vi "SubPanel_DataCollection_Rev11_v8.vi"(0 "DCPowerInformationClusterArray_Input":T2(array[cluster]), 1 "VISAPowerInfoInputArray":T7(array[cluster]), 2 "Run Data SubPanel Input":T6, 3 "RF Block Parameters":T5, 4 "Oscilloscope Info Array":T4(array[cluster]) {"vertical coupling" items=["AC", "DC", "Ground"]}, 6 "New Run?":bool, 7 "error in":errorcluster) -> (16 "data going into the binary file":T1, 20 "DCPowerInformationClusterArray_Output":T2(array[cluster]), 21 "VISAPowerInfoInputOutput":T7(array[cluster]), 22 "Run Data SubPanel Output":T6, 23 "RF Block Parameters Output":T5, 24 "Oscilloscope Info Array Output":T4(array[cluster]) {"vertical coupling" items=["AC", "DC", "Ground"]}, 25 "Reinitialize?":bool, 26 "Data Was Collected?":bool, 27 "error out":errorcluster)   [LabVIEW 2019]
uses:
  Controls/QueueDataControl.ctl
  Controls/DataBlockControl.ctl
  Controls/QueueDataControl_V2.ctl
  <vilib>/Analysis/NI_AALBase.lvlib
  Controls/QueueDataControl_V3.ctl
  <vilib>/Analysis/1siggen.llb/Ramp Pattern by Delta.vi
  <vilib>/Utility/file.llb/Write Delimited Spreadsheet (string).vi
  Controls/RFBlockControl.ctl
  <instrlib>/niScope/Controls/niScope vertical coupling.ctl
panel:
  out "DCPowerInfoArray":string[][](array[string])
  out "Array":string[][][](array[string])
  out "Current Measurements":cluster{dbl[], dbl[]}[](graph)
  out "Voltage Measurements":cluster{dbl[], dbl[]}[](graph)
  out "DCPowerInformationClusterArray_Input 2":T2(array[cluster])
  out "Exiting":bool
  out "Full Run Information":string
  out "Ready For Next Run?":bool
  in  "Next Run":bool
  out "Latchup Output Data":dbl[][](array[numeric])
  out "Recording Data":bool
  out "Current 2":waveform(dbl)[](graph)
  out "Voltage 2":waveform(dbl)[](graph)
  out "Current":waveform(dbl)[](graph)
  out "Voltage":waveform(dbl)[](graph)
  in  "End Collecting":bool
  in  "Record Data Toggle":bool
  out "error of collection":errorcluster
  in  "force exit SubVI":bool
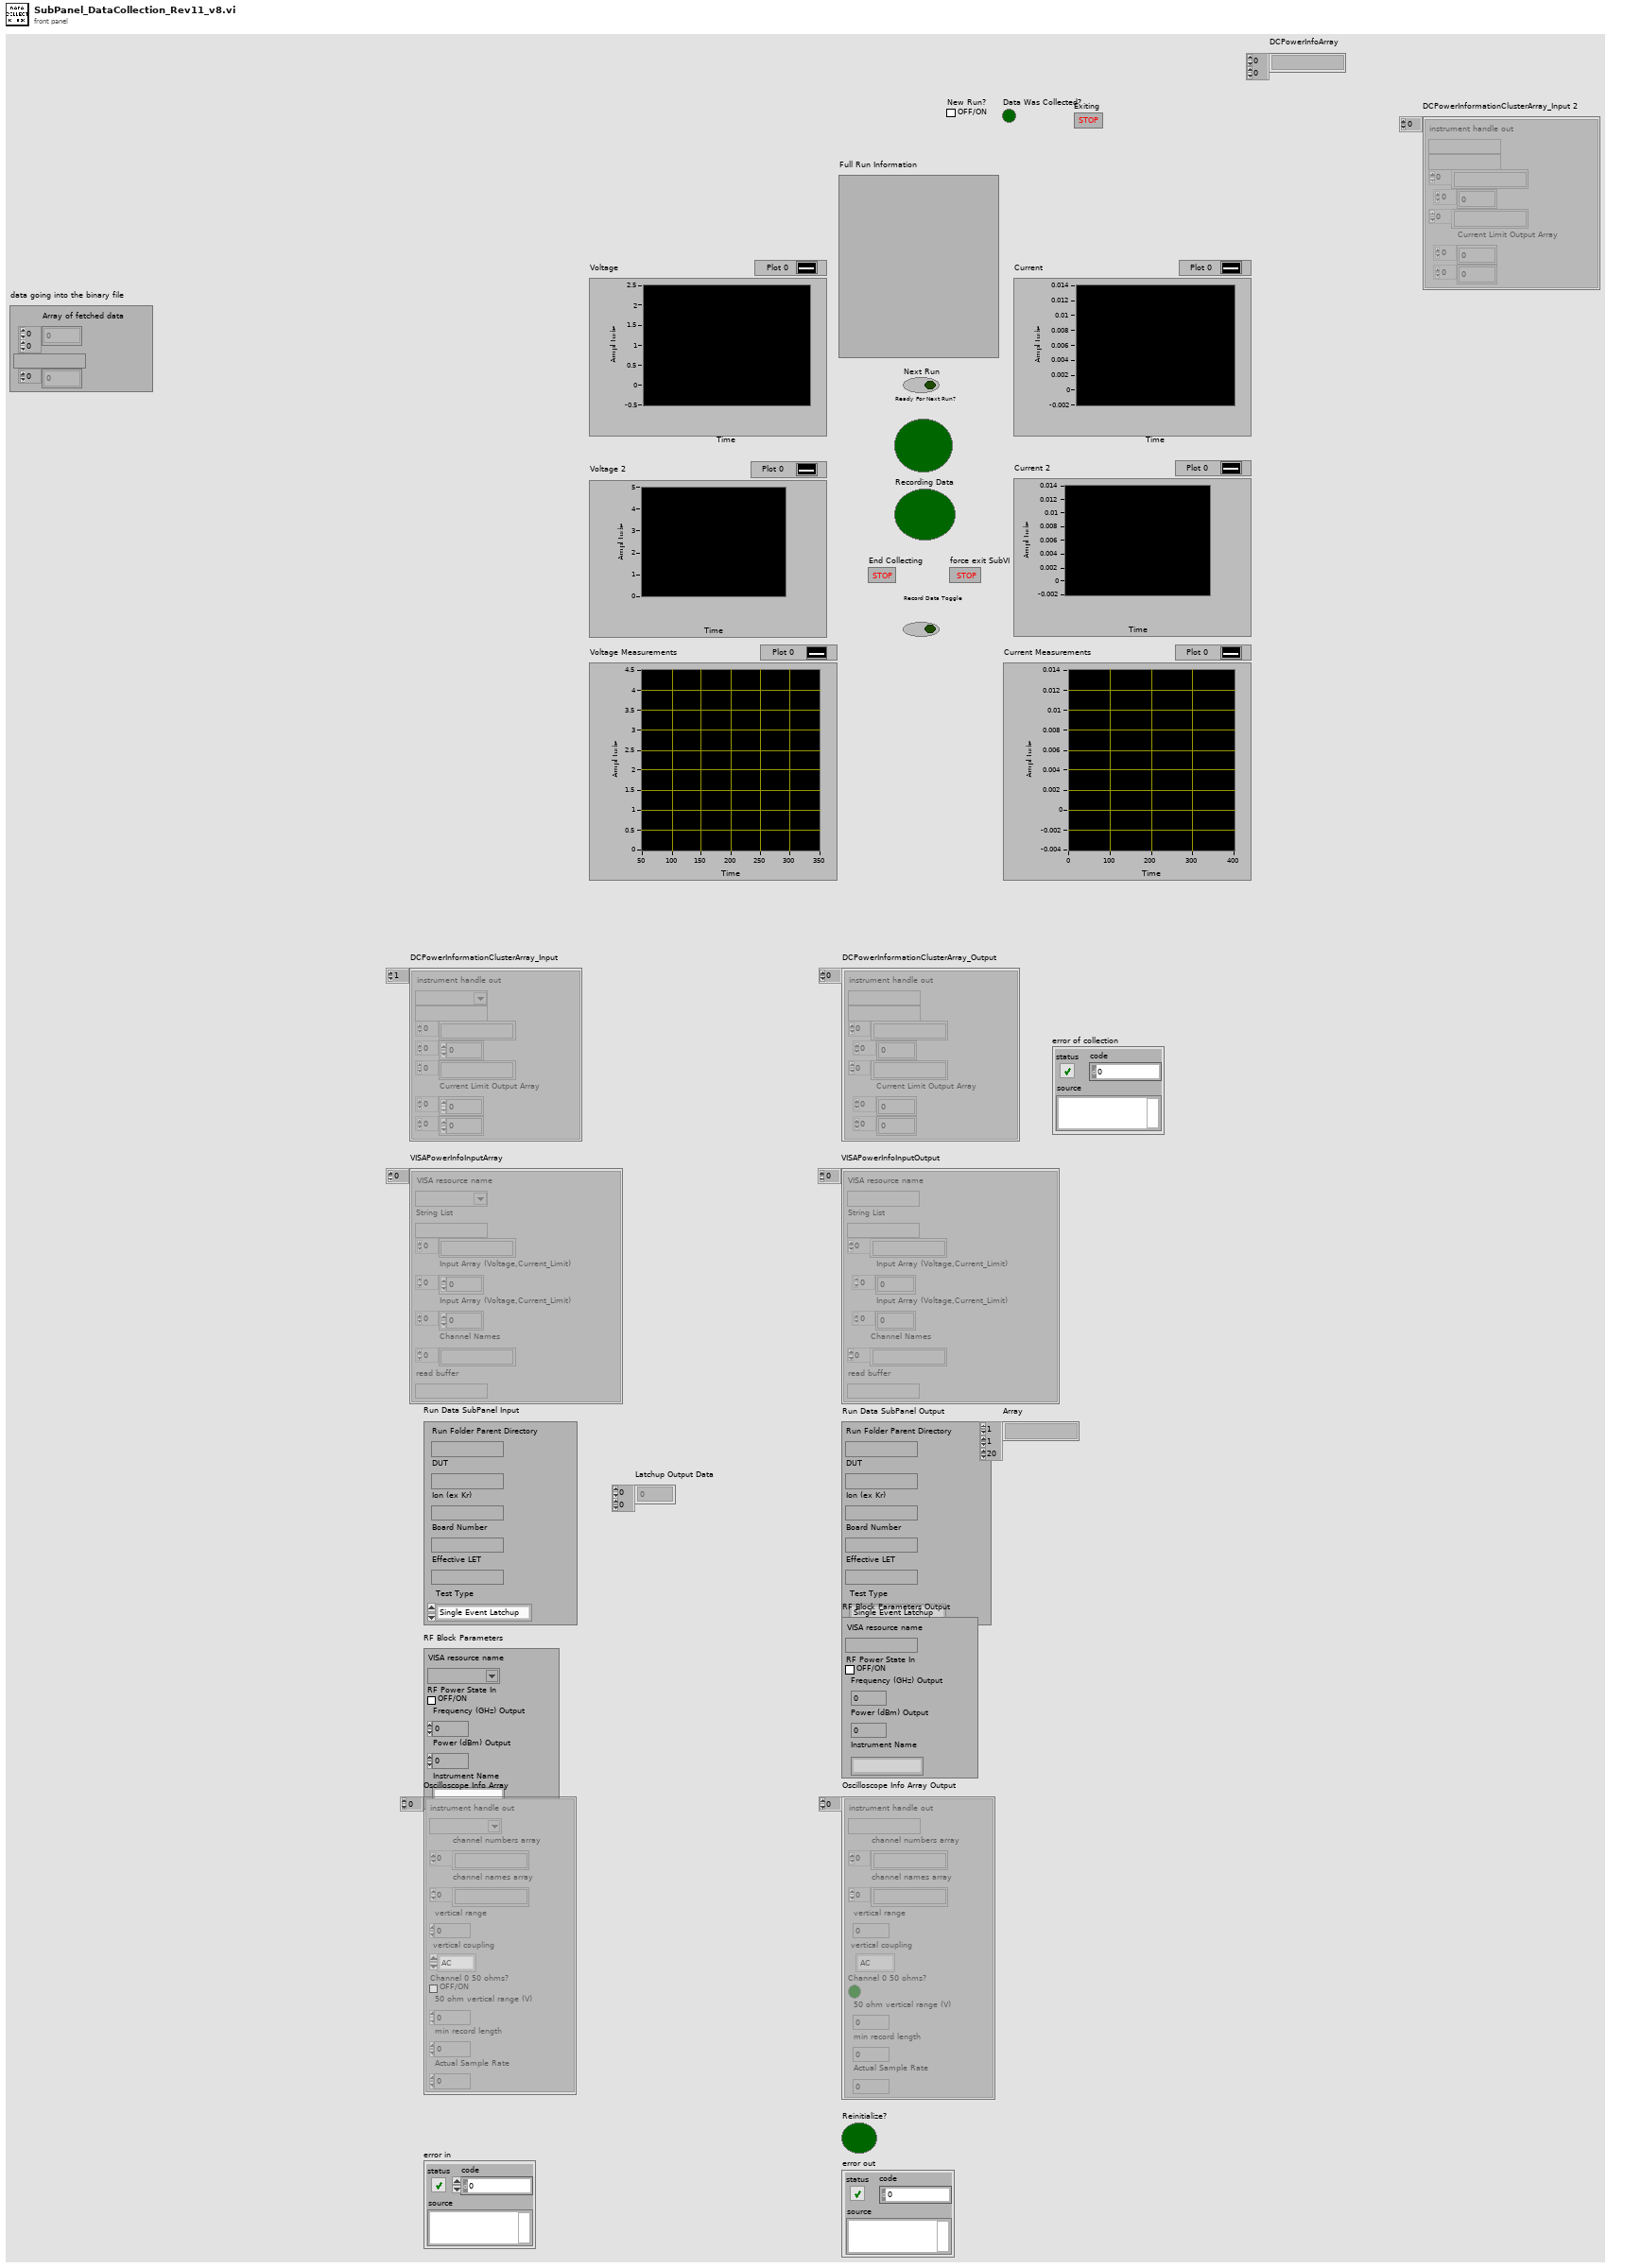
[diagram p1: front panel]
types:
  T1 = cluster{"Array of fetched data":dbl[][], string, i32[]}
  T2 = cluster{"instrument handle out":refnum<k15>, string, string[], dbl[], string[], "Current Limit Output Array":dbl[], dbl[]}[]
  T3 = typedef "niScope vertical coupling.ctl" = i32
  T4 = cluster{"instrument handle out":refnum<k15>, "channel numbers array":string[], "channel names array":string[], "vertical range":dbl, "vertical coupling":T3, "Channel 0 50 ohms?":bool, "50 ohm vertical range (V)":dbl, "min record length":i32, "Actual Sample Rate":dbl}[]
  T5 = typedef "RFBlockControl.ctl" = cluster{"VISA resource name":refnum<visa-resource-name>, "RF Power State In":bool, "Frequency (GHz) Output":dbl, "Power (dBm) Output":dbl, "Instrument Name":string}
  T6 = typedef "DataBlockControl.ctl" = cluster{"Run Folder Parent Directory":path, "DUT":string, "Ion (ex Kr)":string, "Board Number":string, "Effective LET":string, "Test Type":enum16{"Single Event Latchup", "Single Event Transient", "Single Event Upset"}}
  T7 = cluster{"VISA resource name":refnum<visa-resource-name>, "String List":string, string[], "Input Array (Voltage,Current_Limit)":dbl[], "Input Array (Voltage,Current_Limit)":dbl[], "Channel Names":string[], "read buffer":string}[]
  T8 = typedef "QueueDataControl_V3.ctl" = cluster{"Array of fetched data":dbl[][][], "Channel Names Array":string[], "Voltage Waveform Array":waveform(dbl)[], "Current Waveform Array":waveform(dbl)[], "Resetting Time":timestamp, "Beam Logic":dbl}
  T9 = typedef "QueueDataControl_V2.ctl" = cluster{"Time Stamp Array":timestamp[], "Initial Time":timestamp, "dt measurement array":dbl[], "samples per capture":i32[], "voltage measurements":dbl[][], "current measurements":dbl[][]}
  T10 = cluster{"IVI Refnum out":refnum<k15>, string, "voltage level channel 23":dbl, "Channel Name 23":string, "Current Limit":dbl, "Measure Record dt":dbl, string}[]
  T11 = cluster{"created path array":path[], "DCPowerInformation_byChannel":cluster{"IVI Refnum out":refnum<k15>, string, "voltage level channel 23":dbl, "Channel Name 23":string, "Current Limit":dbl, "Measure Record dt":dbl, string}[], string[]}
  T12 = typedef "QueueDataControl.ctl" = cluster{"Rolling Timer":timestamp, "Initial Time":timestamp, "dt between samples":dbl[], "number of samples per fetch":i32[], "voltage measurements":dbl[][], "current measurements":dbl[][]}
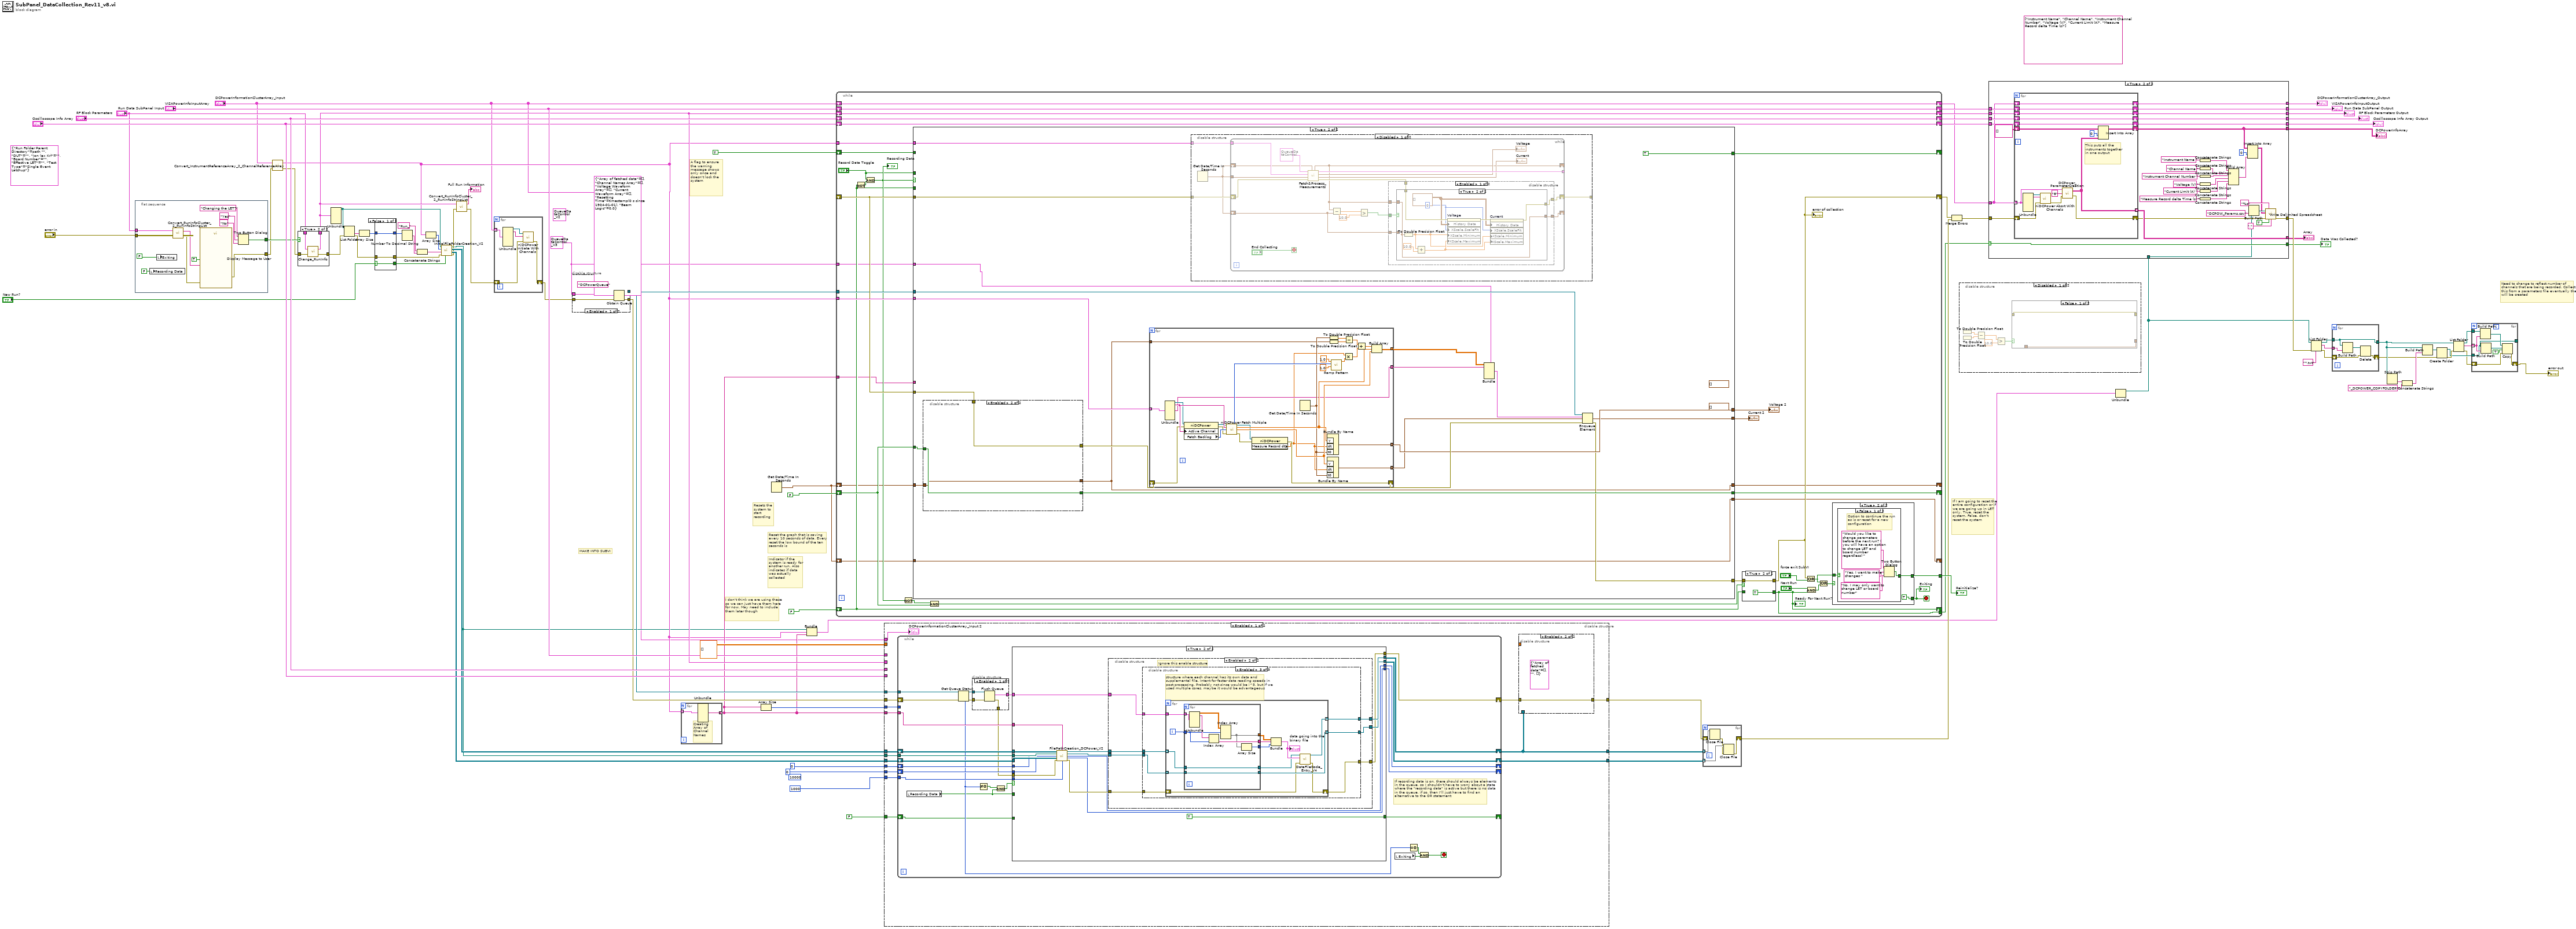
[diagram p0: block diagram]
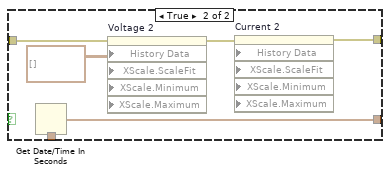
[diagram p2: hidden frame]
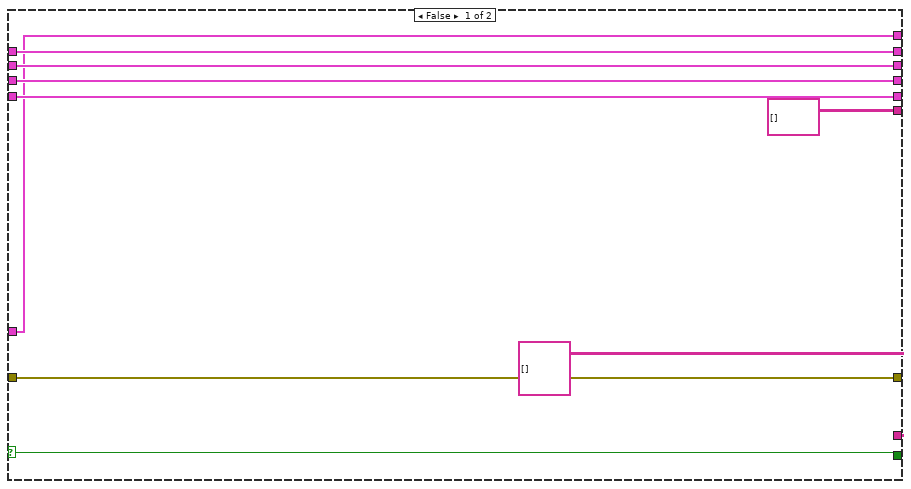
[diagram p4: hidden frame]
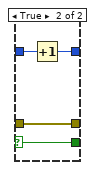
[diagram p5: hidden frame]
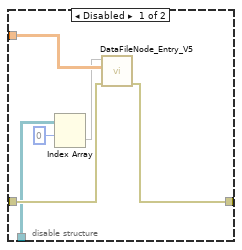
[diagram p8: hidden frame]
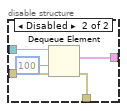
[diagram p9: hidden frame]
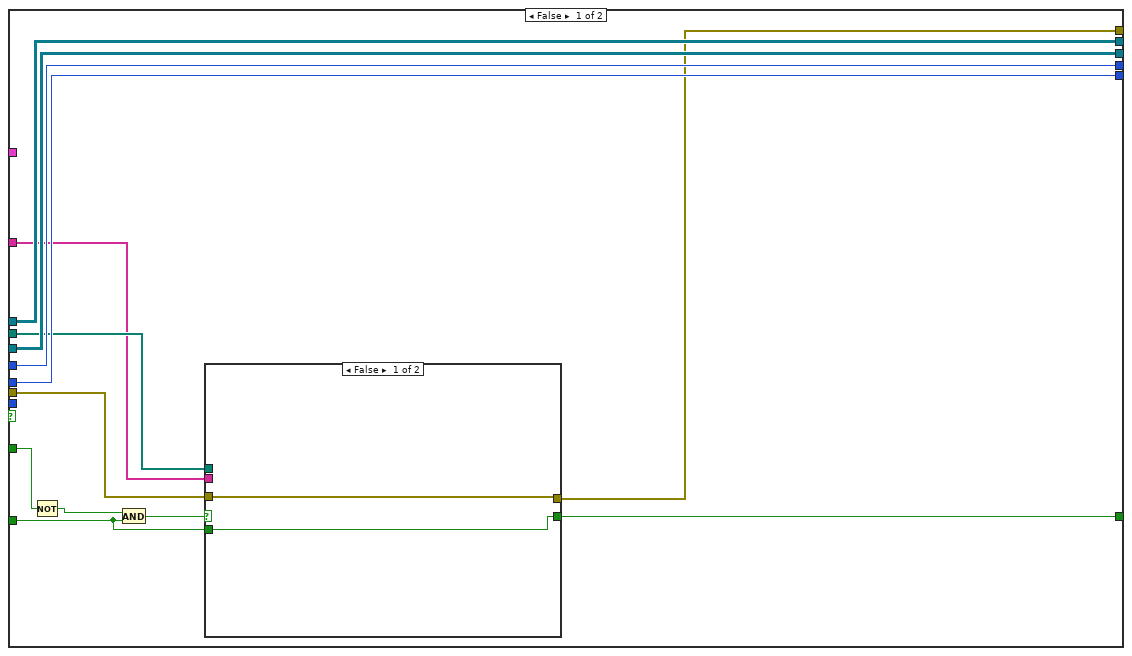
[diagram p10: hidden frame]
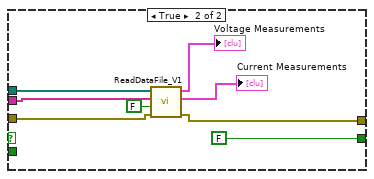
[diagram p11: hidden frame]
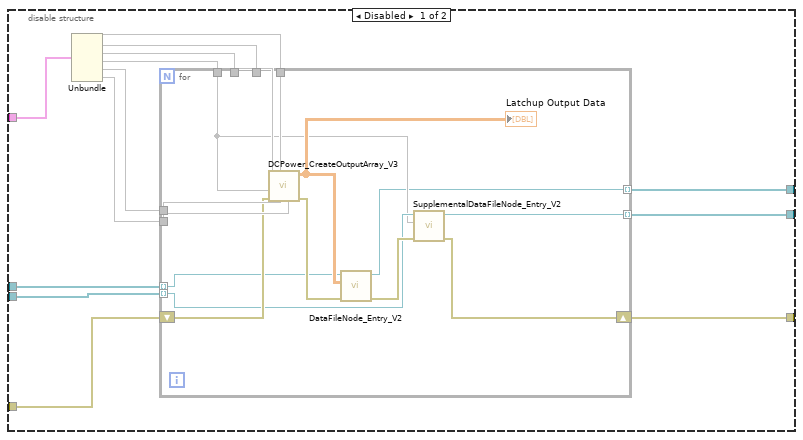
[diagram p12: hidden frame]
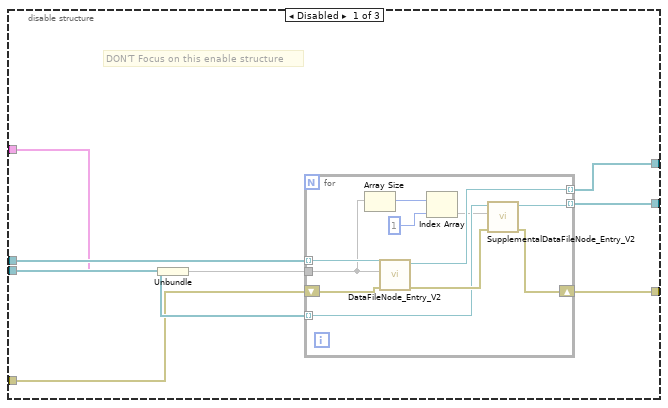
[diagram p13: hidden frame]
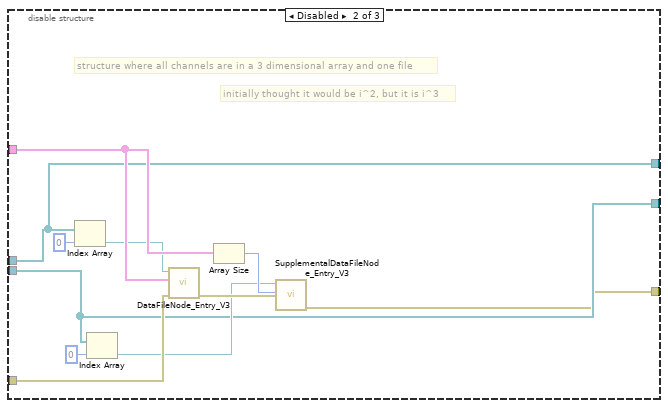
[diagram p14: hidden frame]
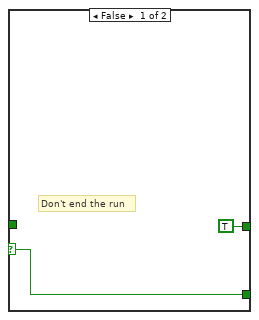
[diagram p16: hidden frame]
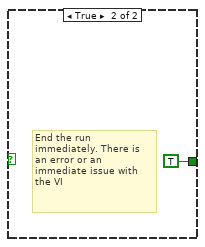
[diagram p17: hidden frame]
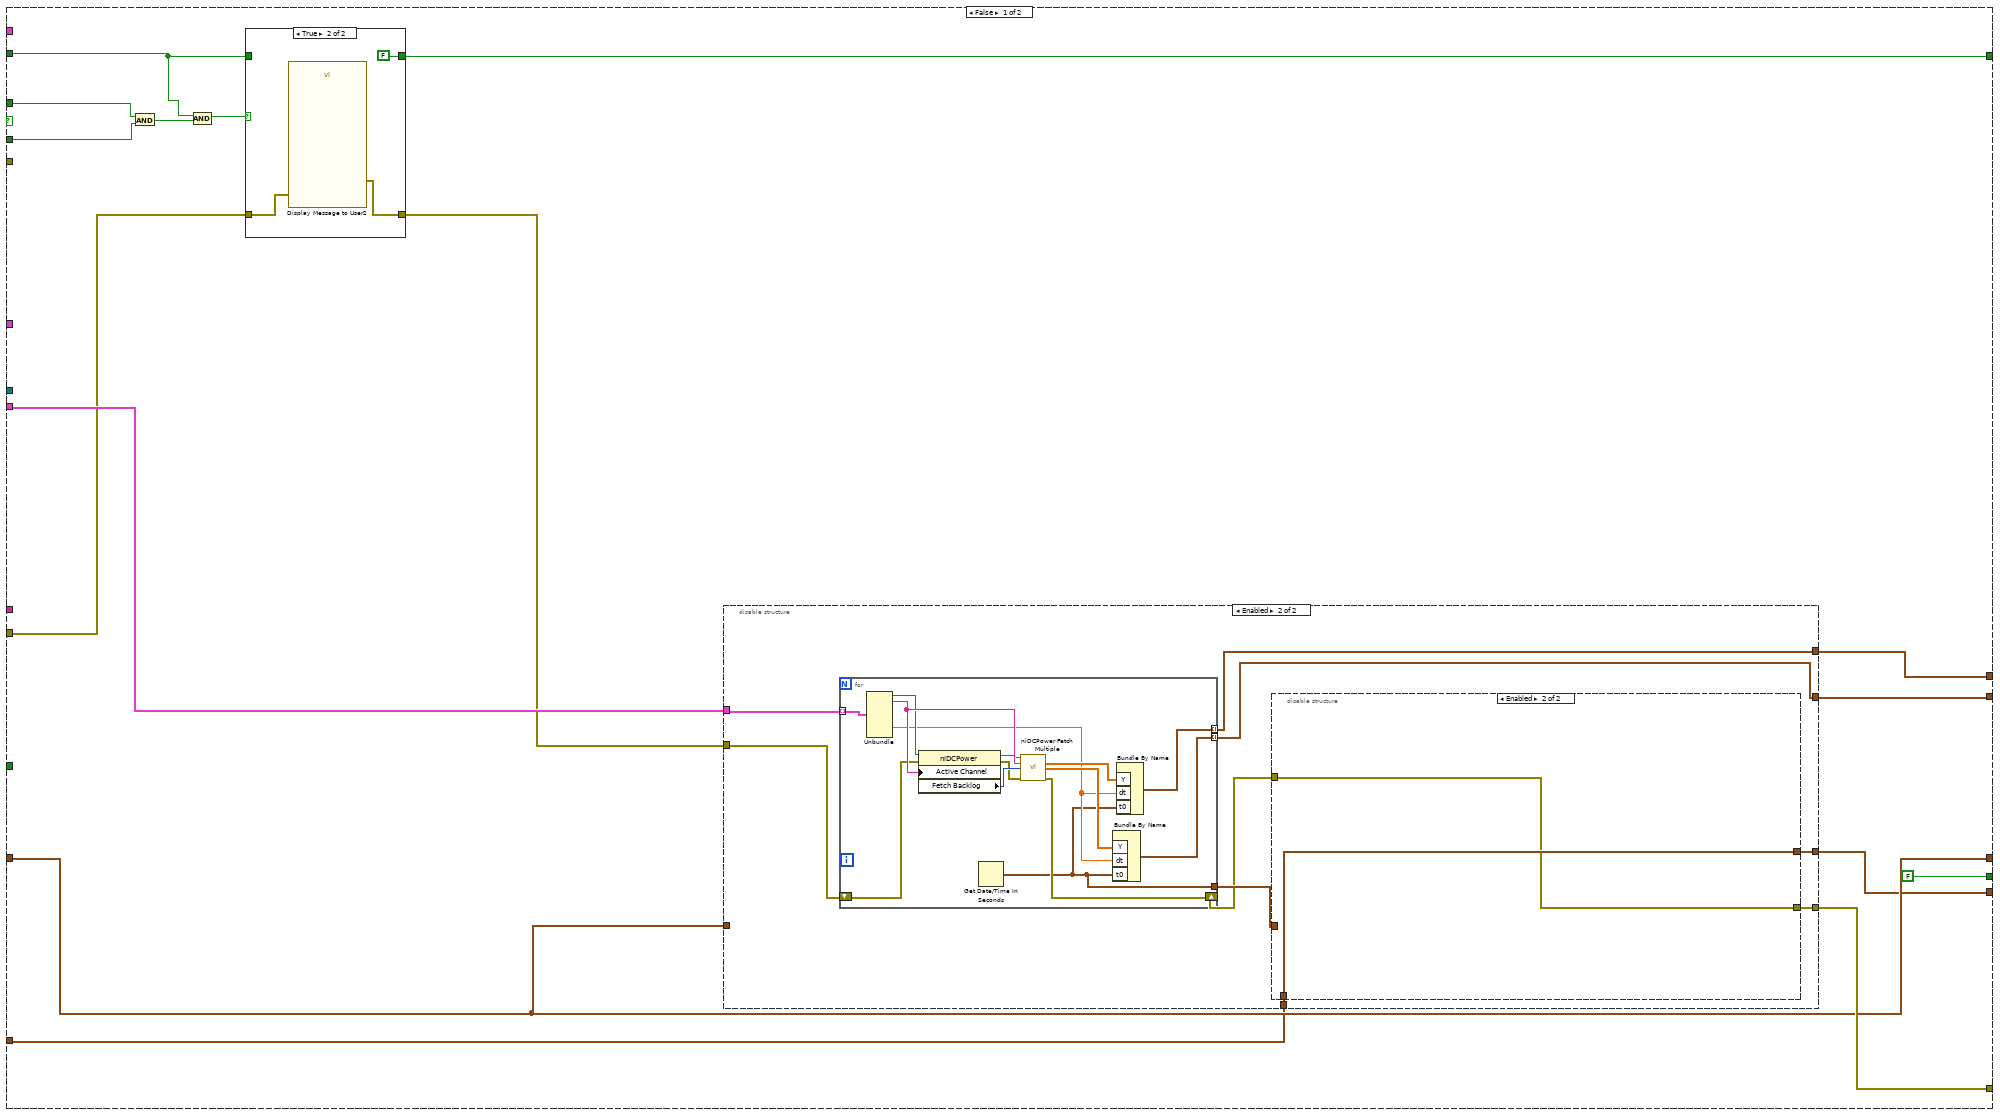
[diagram p19: hidden frame]
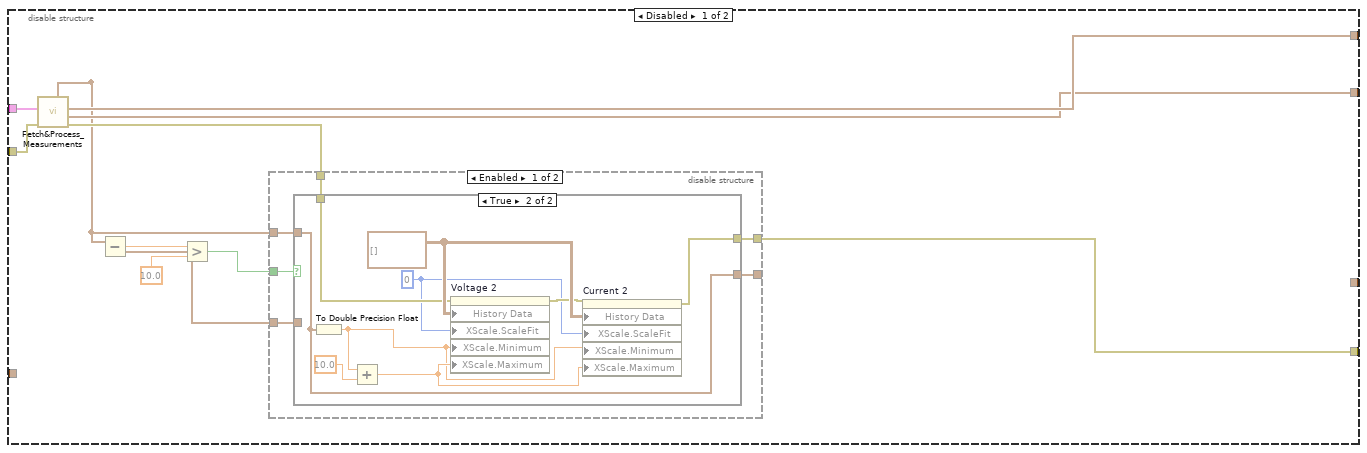
[diagram p20: hidden frame]
diagram:
  (unwired) string[] ["Instrument Name", "Channel Name", "Instrument Channel Number", "Voltage (V)", "Current Limit (A)", "Measure Record delta Time (s)"] ("new element/subarray")
  w50 = T8 {"Array of fetched data"=[], "Channel Names Array"=[], "Voltage Waveform Array"=[], "Current Waveform Array"=[], "Resetting Time"=timestamp(0 s since 1904-01-01), "Beam Logic"=0.0} ("DCPower Queue Data Double Array Format")
  (unwired) T8 {"Array of fetched data"=[], "Channel Names Array"=[], "Voltage Waveform Array"=[], "Current Waveform Array"=[], "Resetting Time"=timestamp(0 s since 1904-01-01), "Beam Logic"=0.0} ("DCPower Double Array Queue")
  (unwired) 10000 ("binary file indexor in")
  (unwired) T9 {"Time Stamp Array"=[], "Initial Time"=timestamp(0 s since 1904-01-01), "dt measurement array"=[], "samples per capture"=[], "voltage measurements"=[], "current measurements"=[]} ("DCPowerDataQueueControl_V2")
  (unwired) T6 {"Run Folder Parent Directory"=path "", "DUT"="", "Ion (ex Kr)"="", "Board Number"="", "Effective LET"="", "Test Type"=enum."Single Event Latchup"} ("Run Data Configuration")
  # "Reset the graph that is saving every 10 seconds of data. Every reset the low bound of the ten seconds is"
  # "Need to change to reflect number of channels that are being recorded. Collect this from a parameters file eventually that will be created"
  # "I don't think we are using these so we can just have them here for now. May need to include them later though"
  # "Indicator if the system is ready for another run. Also indicates if data was actually collected"
  # "Resets the system to start recording"
  # "A flag to ensure the warning message shows only once and doesn't lock the system"
  # "If I am going to reset the entire configuration or if we are going up in LET only. True, reset the system. False, don't reset the system"
  # "MAKE INTO SUBVI"
  n1 = flat-sequence {
    tunnel: [w93] -> w67
    tunnel: "error in" -> [w92]
    tunnel: [w97] -> w75
    tunnel: "Run Data SubPanel Input" -> [w90]
    frame #0 {
      n2 = local write "Recording Data"(FALSE ("Recording Data")) -> ()
      n3 = local write "Exiting"(FALSE ("Forced Exit")) -> ()
      n4 = call "Convert_RunInfoCluster_2_RunInfoStringList.vi"("error in"=w92, "Run Data SubPanel Input"=w90) -> ("error output"=w91:errorcluster, "Run Data Output"=w89:string)
      n5 = call "Display Message to User"("error in (no error)"=w91, "Enable"=TRUE, "Message"=w89) -> ("error out"=w93:errorcluster)  [unwired: 7 in, 1 out]
      n6 = Two Button Dialog(message="Changing the LET?", 1:"No" ("F button name (\"Cancel\")"), 2:"Yes" ("T button name (\"OK\")")) -> (T button?=w97:bool)
    }
  }
  n7 = call "Convert_InstrumentReferenceArray_2_ChannelReferenceArray.vi"("error in (no error)"=w67, "DCPowerInformationClusterArray_Input"="DCPowerInformationClusterArray_Input") -> ("error out"=w66:errorcluster, "DCPowerInformation_byChannel"=w22:T10)
  n8 = case shown="True" w75 {
    tunnel: "Run Data SubPanel Input" -> [w99 w103]
    tunnel: [w99 w102] -> w72
    tunnel: [w98 w101] -> w69
    tunnel: w66 -> [w98 w100]
    frame False {
    }
    frame True {
      n9 = call "Change_RunInfo.vi"("error in (no error)"=w100, "Run Data SubPanel in"=w103) -> ("error out"=w101:errorcluster, "Run Data SubPanel out"=w102:T6)
    }
  }
  n10 = Unbundle(w72) -> ("Run Folder Parent Directory"=w70:path)  [unwired: 5 out]
  n11 = List Folder(path=w70, error in=w69) -> (folder names=w71:string[], error out=w54:errorcluster)  [unwired: 2 in, 2 out]
  n12 = Array Size(array=w71) -> (size(s)=w57:i32)
  n13 = case shown="False" "New Run?" {
    selector: "New Run?" -> [w105 w108]
    tunnel: [w106 w110] -> w58
    tunnel: w57 -> [w106 w109]
    tunnel: [w105 w108] -> w56
    tunnel: [w104 w107] -> w55
    tunnel: w54 -> [w104 w107]
    frame False {
    }
    frame True {
      n14 = Increment(x=w109) -> (x+1=w110:i32)
    }
  }
  n15 = Number To Decimal String(number=w58) -> (decimal integer string=w61:string)  [unwired: 1 in]
  n16 = Concatenate Strings("Run_", w61) -> (w68:string)
  n17 = Array Size(array=w22) -> (size(s)=w53:i32)
  n18 = call "InitialFileFolderCreation_V2.vi"("New Run?"=w56, "error in (no error)"=w55, "Run Number"=w68, "Subfolders&NumChannelsRecorded"=w53, "base path"=w70) -> ("error out"=w52:errorcluster, "SupplementalDataFileReferenceObjectArrayWsubfolders"=w64:refnum<file>[][], "DataFileReferenceObjectArrayWsubfolders"=w65:refnum<file>[][], "created path array"=w6:path[])  [unwired: 3 in]
  n19 = call "Convert_RunInfoCluster_2_RunInfoStringList.vi"("error in"=w52, "Run Data SubPanel Input"=w72) -> ("error output"=w4:errorcluster, "Run Data Output"=→"Full Run Information":string)
  n20 = for {
    shift-right: [w111] -> w3
    shift-left: w4 -> [w113]
    tunnel: "DCPowerInformationClusterArray_Input" -> [w115] mode=indexing
    n21 = Unbundle(w115) -> ("instrument handle out"=w112:refnum<k15>, w114:string)  [unwired: 5 out]
    n22 = call <instrlib>:"niDCPower Initiate With Channels.vi"("error in (no error)"=w113, "channel name"=w114, "instrument handle"=w112) -> ("error out"=w111:errorcluster)  [unwired: 7 in, 1 out]
  }
  n23 = disable-structure shown="Enabled" {
    disable-tunnel: w3 -> [w119 w121]
    disable-tunnel: [w118 w121] -> w80
    disable-tunnel: [w117 _] -> w81
    disable-tunnel: w50 -> [w116 _]
    frame Enabled {
      n24 = Obtain Queue(name (unnamed)="DCPowerQueue", element data type=w116, error in (no error)=w119) -> (queue out=w117:refnum<queue>, error out=w118:errorcluster)  [unwired: 2 in, 1 out]
    }
    frame Disabled {
    }
  }
  n25 = for {
    tunnel: w22 -> [w123] mode=indexing
    tunnel: [w122] -> w23 mode=indexing
    # "Creating Array of Channel Names"
    n26 = Unbundle(w123) -> ("Channel Name 23"=w122:string)  [unwired: 6 out]
  }
  n27 = Array Size(array=w23) -> (size(s)=w44:i32)
  n28 = Get Date/Time In Seconds() -> (seconds since 1Jan1904=w1:timestamp)
  n29 = Bundle("created path array"=w6, "DCPowerInformation_byChannel"=w22, w23) -> (w21:T11)  [unwired: 1 in]
  n30 = while {
    shift-right: [w156] -> w11
    shift-left: "DCPowerInformationClusterArray_Input" -> [w156]
    shift-right: [w160] -> w13
    shift-left: "VISAPowerInfoInputArray" -> [w160]
    shift-right: [w159] -> w15
    shift-left: w72 -> [w159]
    shift-right: [w158] -> w17
    shift-left: "RF Block Parameters" -> [w158]
    shift-right: [w157] -> w19
    shift-left: "Oscilloscope Info Array" -> [w157]
    shift-right: [w140] -> w51
    shift-left: _ -> [w153]
    tunnel: w22 -> [w155]
    tunnel: w22 -> [w154]
    shift-right: [w150] -> _
    shift-left: FALSE -> [w147]
    tunnel: w81 -> [w149]
    shift-right: [w129] -> _
    shift-left: FALSE -> [w134]
    tunnel: [w138] -> w79
    shift-right: [w132] -> _
    shift-left: TRUE ("x .and. y?") -> [w133]
    shift-right: [w130] -> _
    shift-left: w1 -> [w131]
    tunnel: [w129] -> w10
    tunnel: w23 -> [w127]
    tunnel: w50 -> [w126]
    shift-right: [w124] -> _
    shift-left: w1 -> [w125]
    stop <- w128 stop-if-true
    n31 = Not(x=w134) -> (.not. x?=w136:bool)
    n32 = And(x="Record Data Toggle", y=w136) -> (x .and. y?=w137:bool)
    "Recording Data" <- w137
    n33 = Not(x=w137) -> (.not. x?=w148:bool)
    n34 = case shown="True" w137 {
      tunnel: w153 -> [_ w294]
      tunnel: w155 -> [_ w293]
      tunnel: w154 -> [w190 w291]
      tunnel: w153 -> [w187 w289]
      tunnel: [w175 w282] -> w152
      tunnel: [w176 w283] -> w151
      tunnel: w147 -> [_ w286]
      tunnel: [FALSE w287] -> w150
      tunnel: w149 -> [_ w285]
      tunnel: [w188 w281] -> w145
      tunnel: "Record Data Toggle" -> [w184 _]
      tunnel: w134 -> [w185 _]
      tunnel: w133 -> [w180 _]
      tunnel: [w181 TRUE] -> w132
      tunnel: w131 -> [w179 w290]
      tunnel: [w179 w280] -> w130
      tunnel: w127 -> [_ _]
      tunnel: w126 -> [_ w277]
      tunnel: w125 -> [w178 w275]
      tunnel: [w177 w275] -> w124
      frame False {
        n35 = And(x=w184, y=w185) -> (x .and. y?=w183:bool)
        n36 = And(x=w180, y=w183) -> (x .and. y?=w182:bool)
        n37 = case shown="True" w182 {
          tunnel: [w271 w273] -> w186
          tunnel: w187 -> [w271 w274]
          tunnel: [w270 FALSE] -> w181
          tunnel: w180 -> [w270 _]
          frame False {
          }
          frame True {
            n38 = call "Display Message to User2"("error in (no error)"=w274) -> ("error out"=w273:errorcluster)  [unwired: 9 in, 1 out]
          }
        }
        n39 = disable-structure shown="Enabled" {
          disable-tunnel: w190 -> [w200 w232]
          disable-tunnel: [w195 w231] -> w176
          disable-tunnel: [w194 w229] -> w175
          disable-tunnel: [w192 w224] -> w188
          disable-tunnel: w186 -> [w191 w230]
          disable-tunnel: w179 -> [_ _]
          disable-tunnel: w178 -> [_ w226]
          disable-tunnel: [_ w225] -> w177
          frame Disabled {
            n40 = call "Fetch&Process_Measurements.vi"("error in (no error)"=w191, "DCPowerInformation_byChannel"=w200) -> ("error out"=w201:errorcluster, "Current Measurement"=w194:waveform(dbl)[], "Voltage Measurement"=w195:waveform(dbl)[], "Rolling Timer Output"=w193:timestamp, "Rolling Timer Input"=w198:timestamp, "Queue Data Parameters in"=w199:T12)  [unwired: 3 in, 1 out]
            n41 = Subtract(x=w193, y=w196) -> (x-y=w203:dbl)
            n42 = Greater?(x=w203, y=10.0) -> (0:w202:bool)
            n43 = disable-structure shown="Enabled" {
              disable-tunnel: w202 -> [w210 _]
              disable-tunnel: w201 -> [w209 w223]
              disable-tunnel: [w208 w223] -> w192
              disable-tunnel: [w207 w222] -> w197
              disable-tunnel: w193 -> [w206 w222]
              disable-tunnel: [w205 _] -> w196
              frame Enabled {
                n44 = case shown="True" w210 {
                  tunnel: w209 -> [w212 w218]
                  tunnel: [w212 w216] -> w208
                  tunnel: [w211 w220] -> w207
                  tunnel: w206 -> [_ w220]
                  tunnel: w205 -> [w211 _]
                  frame False {
                  }
                  frame True {
                    w215 = u8 0 ("X Scale.Scale Fit")
                    w219 = waveform(dbl)[][] [] ("History Data")
                    n45 = To Double Precision Float(number=w220) -> (double precision float=w213:dbl)
                    n46 = Add(x=w213, y=10.0) -> (x+y=w214:dbl)
                    n47 = property on="Voltage 2" class="WFChart (strict)"(error in=w218, "History Data"=w219, "XScale.ScaleFit"=w215, "XScale.Minimum"=w213, "XScale.Maximum"=w214) -> (error out=w217:errorcluster)  [unwired: 1 in, 1 out]
                    n48 = property on="Current 2" class="WFChart (strict)"(error in=w217, "History Data"=w219, "XScale.ScaleFit"=w215, "XScale.Minimum"=w213, "XScale.Maximum"=w214) -> (error out=w216:errorcluster)  [unwired: 1 in, 1 out]
                  }
                }
              }
              frame Disabled {
              }
            }
          }
          frame Enabled {
            n49 = for {
              tunnel: w232 -> [w269] mode=indexing
              tunnel: [w262] -> w231 mode=indexing
              tunnel: [w261] -> w229 mode=indexing
              shift-right: [w258] -> w227
              shift-left: w230 -> [w266]
              tunnel: [w256] -> w228
              n50 = Unbundle(w269) -> ("IVI Refnum out"=w265:refnum<k15>, w268:string, "Measure Record dt"=w257:dbl)  [unwired: 4 out]
              n51 = property class="niDCPower"(reference=w265, error in=w266, "Active Channel"=w268) -> (reference out=w264:refnum<k15>, error out=w263:errorcluster, "Fetch Backlog"=w267:i32)
              n52 = Get Date/Time In Seconds() -> (seconds since 1Jan1904=w256:timestamp)
              n53 = call <instrlib>:"niDCPower Fetch Multiple.vi"("instrument handle"=w264, "channel name"=w268, "count (1)"=w267, "error in (no error)"=w263) -> ("voltage measurements"=w259:dbl[], "current measurements"=w260:dbl[], "error out"=w258:errorcluster)  [unwired: 6 in, 3 out]
              n54 = Bundle By Name("Y"=w260, "dt"=w257, "t0"=w256) -> (w261:waveform(dbl))  [unwired: 1 out]
              n55 = Bundle By Name("Y"=w259, "dt"=w257, "t0"=w256) -> (w262:waveform(dbl))  [unwired: 1 out]
            }
            n56 = disable-structure shown="Enabled" {
              disable-tunnel: w228 -> [w240 _]
              disable-tunnel: w227 -> [w236 w254]
              disable-tunnel: w226 -> [w235 w255]
              disable-tunnel: [w234 w255] -> w225
              disable-tunnel: [w233 w254] -> w224
              frame Disabled {
                n57 = To Double Precision Float(number=w240) -> (double precision float=w241:dbl)
                n58 = To Double Precision Float(number=w235) -> (double precision float=w242:dbl)
                n59 = Subtract(x=w241, y=w242) -> (x-y=w239:dbl)
                n60 = Greater?(x=w239, y=10.0) -> (0:w237:bool)
                n61 = case shown="True" w237 {
                  tunnel: w236 -> [w243 w253]
                  tunnel: [w244 w250] -> w234
                  tunnel: w235 -> [w244 _]
                  tunnel: [w243 w251] -> w233
                  frame False {
                  }
                  frame True {
                    w249 = u8 0 ("X Scale.Scale Fit")
                    w248 = waveform(dbl)[][] [] ("History Data")
                    n62 = Get Date/Time In Seconds() -> (seconds since 1Jan1904=w250:timestamp)
                    n63 = To Double Precision Float(number=w250) -> (double precision float=w246:dbl)
                    n64 = Add(x=10.0, y=w246) -> (x+y=w245:dbl)
                    n65 = property on="Voltage 2" class="WFChart (strict)"(error in=w253, "History Data"=w248, "XScale.ScaleFit"=w249, "XScale.Minimum"=w246, "XScale.Maximum"=w245) -> (error out=w252:errorcluster)  [unwired: 1 in, 1 out]
                    n66 = property on="Current 2" class="WFChart (strict)"(error in=w252, "History Data"=w248, "XScale.ScaleFit"=w249, "XScale.Minimum"=w246, "XScale.Maximum"=w245) -> (error out=w251:errorcluster)  [unwired: 1 in, 1 out]
                  }
                }
              }
              frame Enabled {
              }
            }
          }
        }
      }
      frame True {
        (unwired) waveform(dbl)[] [] ("array")
        (unwired) waveform(dbl)[] []
        n67 = disable-structure shown="Enabled" {
          disable-tunnel: w290 -> [w300 w314]
          disable-tunnel: w289 -> [w299 w316]
          disable-tunnel: [w298 w316] -> w288
          disable-tunnel: [w297 w315] -> w287
          disable-tunnel: w286 -> [w296 w315]
          disable-tunnel: [w295 w314] -> w280
          frame Disabled {
            n68 = case shown="False" w296 {
              tunnel: [w305 w313] -> w295
              tunnel: w300 -> [_ w313]
              tunnel: w299 -> [w310 w312]
              tunnel: [w308 w312] -> w298
              tunnel: [TRUE w311] -> w297
              tunnel: w296 -> [_ w311]
              frame False {
                w301 = waveform(dbl)[][] [] ("History Data")
                w306 = u8 0 ("X Scale.Scale Fit")
                n69 = Get Date/Time In Seconds() -> (seconds since 1Jan1904=w305:timestamp)
                n70 = To Double Precision Float(number=w305) -> (double precision float=w302:dbl)
                n71 = Add(x=10.0 ("y"), y=w302) -> (x+y=w304:dbl)
                n72 = property on="Voltage 2" class="WFChart (strict)"(error in=w310, "History Data"=w301, "XScale.ScaleFit"=w306, "XScale.Minimum"=w302, "XScale.Maximum"=w304) -> (error out=w309:errorcluster)  [unwired: 1 in, 1 out]
                n73 = property on="Current 2" class="WFChart (strict)"(error in=w309, "History Data"=w301, "XScale.ScaleFit"=w306, "XScale.Minimum"=w302, "XScale.Maximum"=w304) -> (error out=w308:errorcluster)  [unwired: 1 in, 1 out]
              }
              frame True {
              }
            }
          }
          frame Enabled {
          }
        }
        n74 = for {
          tunnel: w291 -> [w344] mode=indexing
          tunnel: [w337] -> w283 mode=indexing
          tunnel: [w336] -> w282 mode=indexing
          shift-right: [w318] -> w284
          shift-left: w288 -> [w341]
          tunnel: w280 -> [w323]
          tunnel: [w322] -> w279 mode=indexing
          tunnel: [w321] -> w278 mode=indexing
          n75 = Unbundle(w344) -> ("IVI Refnum out"=w340:refnum<k15>, w343:string, "Channel Name 23"=w321:string)  [unwired: 4 out]
          n76 = property class="niDCPower"(reference=w340, error in=w341, "Active Channel"=w343) -> (reference out=w339:refnum<k15>, error out=w338:errorcluster, "Fetch Backlog"=w342:i32)
          n77 = call <instrlib>:"niDCPower Fetch Multiple.vi"("instrument handle"=w339, "channel name"=w343, "count (1)"=w342, "error in (no error)"=w338) -> ("actual count"=w325:i32, "instrument handle out"=w320:refnum<k15>, "voltage measurements"=w327:dbl[], "current measurements"=w326:dbl[], "error out"=w319:errorcluster)  [unwired: 6 in, 1 out]
          n78 = property class="niDCPower"(reference=w320, error in=w319) -> (error out=w318:errorcluster, "Measure Record dt"=w317:dbl)  [unwired: 1 out]
          n79 = Get Date/Time In Seconds() -> (seconds since 1Jan1904=w324:timestamp)
          n80 = Bundle By Name("Y"=w327, "dt"=w317, "t0"=w324) -> (w337:waveform(dbl))  [unwired: 1 out]
          n81 = Bundle By Name("Y"=w326, "dt"=w317, "t0"=w324) -> (w336:waveform(dbl))  [unwired: 1 out]
          n82 = To Double Precision Float(number=w324) -> (double precision float=w333:dbl)
          n83 = To Double Precision Float(number=w323) -> (double precision float=w332:dbl)
          n84 = call-poly <vilib>:"Ramp Pattern.vi"("start"=1.0, "end"=w325, "delta"=1.0) -> ("Ramp Pattern"=w329:dbl[])  [unwired: 6 in, 2 out]
          n85 = Multiply(x=w317, y=w329) -> (x*y=w328:dbl[])
          n86 = Subtract(x=w333, y=w332) -> (x-y=w330:dbl)
          n87 = Add(x=w330, y=w328) -> (x+y=w335:dbl[])
          n88 = Build Array(w335, w327, w326) -> (w322:dbl[][])
        }
        n89 = disable-structure shown="Disabled" {
          disable-tunnel: w294 -> [w348 _]
          disable-tunnel: w293 -> [w347 _]
          disable-tunnel: [w346 errorcluster {"status"=FALSE, "code"=0, "source"=""} ("error out")] -> _
          frame Disabled {
            n90 = Get Date/Time In Seconds() -> (seconds since 1Jan1904=w345:timestamp)
            n91 = while {
              shift-right: [w352] -> w346
              shift-left: w348 -> [w363]
              tunnel: w347 -> [w364]
              tunnel: w345 -> [w360]
              shift-right: [w350] -> _
              shift-left: w345 -> [w361]
              tunnel: [w359] -> _
              shift-right: [w351] -> _
              shift-left: w345 -> [w349]
              stop <- "End Collecting" stop-if-true
              n92 = call "Fetch&Process_Measurements.vi"("Rolling Timer Input"=w361, "error in (no error)"=w363, "Initial Time"=w360, "DCPowerInformation_byChannel"=w364, "Queue Data Parameters in"=T12 {"Rolling Timer"=timestamp(0 s since 1904-01-01), "Initial Time"=timestamp(0 s since 1904-01-01), "dt between samples"=[], "number of samples per fetch"=[], "voltage measurements"=[], "current measurements"=[]} ("Queue Data Parameters")) -> ("error out"=w353:errorcluster, "Current Measurement"=→"Current":waveform(dbl)[], "Voltage Measurement"=→"Voltage":waveform(dbl)[], "Queue Data Parameters out"=w359:T12, "Rolling Timer Output"=w350:timestamp)  [unwired: 2 in]
              n93 = Subtract(x=w350, y=w349) -> (x-y=w355:dbl)
              n94 = Greater?(x=w355, y=10.0) -> (0:w354:bool)
              n95 = disable-structure shown="Enabled" {
                disable-tunnel: w354 -> [w371 _]
                disable-tunnel: w353 -> [w370 w384]
                disable-tunnel: [w369 w384] -> w352
                disable-tunnel: [w368 w383] -> w351
                disable-tunnel: w350 -> [w367 w383]
                disable-tunnel: w349 -> [w366 _]
                frame Enabled {
                  n96 = case shown="True" w371 {
                    tunnel: w370 -> [w373 w382]
                    tunnel: [w373 w380] -> w369
                    tunnel: [w372 w374] -> w368
                    tunnel: w367 -> [_ w374]
                    tunnel: w366 -> [w372 _]
                    frame False {
                    }
                    frame True {
                      w377 = u8 0 ("X Scale.Scale Fit")
                      w378 = waveform(dbl)[][] [] ("History Data")
                      n97 = To Double Precision Float(number=w374) -> (double precision float=w375:dbl)
                      n98 = Add(x=w375, y=10.0) -> (x+y=w376:dbl)
                      n99 = property on="Voltage" class="WFChart (strict)"(error in=w382, "History Data"=w378, "XScale.ScaleFit"=w377, "XScale.Minimum"=w375, "XScale.Maximum"=w376) -> (error out=w381:errorcluster)  [unwired: 1 in, 1 out]
                      n100 = property on="Current" class="WFChart (strict)"(error in=w381, "History Data"=w378, "XScale.ScaleFit"=w377, "XScale.Minimum"=w375, "XScale.Maximum"=w376) -> (error out=w380:errorcluster)  [unwired: 1 in, 1 out]
                    }
                  }
                }
                frame Disabled {
                }
              }
            }
          }
          frame Enabled {
          }
        }
        n101 = Bundle(cluster=w277, "Array of fetched data"=w279, "Channel Names Array"=w278) -> (w276:T8)  [unwired: 4 in]
        n102 = Enqueue Element(queue=w285, element=w276, error in (no error)=w284) -> (error out=w281:errorcluster)  [unwired: 1 in, 2 out]
      }
    }
    "Voltage 2" <- w151
    "Current 2" <- w152
    n103 = And(x=w148, y=w147) -> (x .and. y?=w146:bool)
    n104 = case shown="True" w146 {
      tunnel: w145 -> [w171 w173]
      tunnel: [w172 TRUE] -> w129
      tunnel: w134 -> [w172 _]
      tunnel: [w171 w173] -> w140
      frame False {
      }
      frame True {
      }
    }
    "error of collection" <- w140
    "Ready For Next Run?" <- w129
    n105 = Or(x=w140, y="force exit SubVI") -> (x .or. y?=w142:bool)
    n106 = And(x="Next Run", y=w129) -> (x .and. y?=w144:bool)
    n107 = Or(x=w142, y=w144) -> (x .or. y?=w143:bool)
    n108 = case shown="True" w143 {
      selector: w143 -> [w162 _]
      tunnel: w142 -> [_ w165]
      tunnel: [w162 TRUE] -> w128
      tunnel: [TRUE ("T button?") w163] -> w138
      frame False {
        # "Don't end the run"
      }
      frame True {
        n109 = case shown="False" w165 {
          tunnel: [w166 TRUE] -> w163
          frame False {
            # "Option to continue the run as is or reset for a new configuration"
            n110 = Two Button Dialog(message="Would you like to change parameters before the next run? ( you will have an option to change LET and board number regardless) ", 1:"No, I may only want to change LET or board number" ("F button name (\"Cancel\")"), 2:"Yes, I want to make changes " ("T button name (\"OK\")")) -> (T button?=w166:bool)
          }
          frame True {
            # "End the run immediately. There is an error or an immediate issue with the VI"
          }
        }
      }
    }
    "Exiting" <- w128
  }
  "Reinitialize?" <- w79
  n111 = disable-structure shown="Enabled" {
    disable-tunnel: "DCPowerInformationClusterArray_Input" -> [w392 _]
    disable-tunnel: "VISAPowerInfoInputArray" -> [_ _]
    disable-tunnel: w72 -> [_ _]
    disable-tunnel: "RF Block Parameters" -> [_ _]
    disable-tunnel: "Oscilloscope Info Array" -> [_ _]
    disable-tunnel: w81 -> [w401 _]
    disable-tunnel: w80 -> [w400 _]
    disable-tunnel: w23 -> [w399 _]
    disable-tunnel: w6 -> [w398 _]
    disable-tunnel: w65 -> [w397 _]
    disable-tunnel: w64 -> [w396 _]
    disable-tunnel: 0 ("binary file indexor in") -> [w395 _]
    disable-tunnel: 0 ("binary file indexor in") -> [w394 _]
    disable-tunnel: 1000 ("binary file indexor in") -> [w393 _]
    disable-tunnel: [w389 _] -> w47
    disable-tunnel: [w388 _] -> w49
    disable-tunnel: [w391 _] -> w48
    disable-tunnel: dbl[][][] [] -> [_ _]
    disable-tunnel: w44 -> [w387 _]
    disable-tunnel: FALSE -> [w386 _]
    frame Enabled {
      n112 = while {
        tunnel: w401 -> [w435]
        shift-right: [w422] -> w390
        shift-left: w400 -> [w434]
        tunnel: w398 -> [w431]
        shift-right: [w424] -> w388
        shift-left: w397 -> [w432]
        shift-right: [w423] -> w391
        shift-left: w396 -> [w430]
        shift-right: [w426] -> _
        shift-left: w395 -> [w429]
        shift-right: [w425] -> _
        shift-left: w394 -> [w428]
        tunnel: w393 -> [w427]
        tunnel: w399 -> [w433]
        tunnel: w387 -> [_]
        shift-right: [w411] -> _
        shift-left: w386 -> [w410]
        stop <- w419 stop-if-true
        # "If recording data is on, there should always be elements in the queue, so I shouldn't have to worry about a state where the \"recording data\" is active but there is no data in the queue, if so, then I'll just have to find an alternative to the OR statement"
        n113 = local read "Recording Data"() -> (w409:bool)
        n114 = Get Queue Status(queue=w435, error in (no error)=w434) -> (queue out=w416:refnum<queue>, error out=w417:errorcluster, # elements in queue=w412:i32)  [unwired: 1 in, 5 out]
        n115 = disable-structure shown="Enabled" {
          disable-tunnel: [w439 w441] -> w418
          disable-tunnel: w417 -> [w438 w443]
          disable-tunnel: w416 -> [w437 w444]
          disable-tunnel: [w436 w440] -> w415
          frame Enabled {
            n116 = Flush Queue(queue=w437, error in (no error)=w438) -> (remaining elements=w436:T8[], error out=w439:errorcluster)  [unwired: 1 out]
          }
          frame Disabled {
            n117 = Dequeue Element(queue=w444, timeout in ms (-1)=100, error in (no error)=w443) -> (element=w440:T8, error out=w441:errorcluster)  [unwired: 2 out]
          }
        }
        n118 = Not Equal To 0?(x=w412) -> (x != 0?=w414:bool)
        n119 = And(x=w414, y=w409) -> (x .and. y?=w413:bool)
        n120 = case shown="True" w413 {
          tunnel: w415 -> [_ w485]
          tunnel: w418 -> [w448 w479]
          tunnel: w433 -> [w449 w471]
          tunnel: w432 -> [w456 w484]
          tunnel: w431 -> [w450 w483]
          tunnel: w430 -> [w457 w482]
          tunnel: w429 -> [w455 w481]
          tunnel: w428 -> [w454 w470]
          tunnel: w427 -> [_ w469]
          tunnel: [w455 w478] -> w426
          tunnel: [w454 w477] -> w425
          tunnel: [w456 w474] -> w424
          tunnel: [w457 w473] -> w423
          tunnel: [w447 w472] -> w422
          tunnel: [w446 TRUE] -> w411
          tunnel: w410 -> [w445 _]
          tunnel: w409 -> [w453 _]
          frame False {
            n121 = Not(x=w453) -> (.not. x?=w452:bool)
            n122 = And(x=w452, y=w445) -> (x .and. y?=w451:bool)
            n123 = case shown="False" w451 {
              tunnel: w450 -> [_ w467]
              tunnel: w449 -> [_ w466]
              tunnel: w448 -> [w459 w464]
              tunnel: [w459 w463] -> w447
              tunnel: [w458 FALSE] -> w446
              tunnel: w445 -> [w458 _]
              frame False {
              }
              frame True {
                n124 = call "ReadDataFile_V1.vi"("error in (no error)"=w464, "Create CSV files?"=FALSE, "Channel Names Array"=w466, "DataFolder Path"=w467) -> ("error out"=w463:errorcluster, "Current Measurements"=→"Current Measurements":cluster{dbl[], dbl[]}[], "Voltage Measurements"=→"Voltage Measurements":cluster{dbl[], dbl[]}[])  [unwired: 5 in]
              }
            }
          }
          frame True {
            n125 = call "FilePathCreation_DCPower_V2.vi"("binary file input reference array 1"=w484, "Channel Name Input array"=w471, "data output directory folder"=w483, "binary file indexor in"=w481, "Reset counter in"=w470, "error in (no error)"=w479, "binary file input reference array 2"=w482, "reset threshold"=w469) -> ("binary file output reference array"=w476:refnum<file>[], "binary file output reference array 2"=w475:refnum<file>[], "binary file indexor out"=w478:i32, "reset counter out"=w477:i32, "error out"=w480:errorcluster)  [unwired: 3 in]
            n126 = disable-structure shown="Enabled" {
              disable-tunnel: w485 -> [w498 w514]
              disable-tunnel: w480 -> [w497 w518]
              disable-tunnel: w476 -> [w496 w520]
              disable-tunnel: w475 -> [w495 w519]
              disable-tunnel: [w494 w517] -> w474
              disable-tunnel: [w493 w516] -> w473
              disable-tunnel: [w492 w515] -> w472
              frame Disabled {
                n127 = Unbundle(w498) -> (w486, w487, w491, w490, w489, w488)
                n128 = for {
                  tunnel: w491 -> [w511]
                  tunnel: w490 -> [w501]
                  tunnel: w489 -> [w510]
                  tunnel: w488 -> [w509]
                  tunnel: w487 -> [w512]
                  tunnel: w486 -> [w513]
                  shift-right: [w503] -> w492
                  shift-left: w497 -> [w508]
                  tunnel: w496 -> [w505] mode=indexing
                  tunnel: w495 -> [w502] mode=indexing
                  tunnel: [w500] -> w494 mode=indexing
                  tunnel: [w499] -> w493 mode=indexing
                  n129 = call "DCPower_CreateOutputArray_V3.vi"("current measurements"=w509, "voltage measurements"=w510, "Time Stamp Array"=w513, "error in"=w508, "actual count"=w501, "Measure Record dt"=w511, "Initial Time"=w512) -> ("error out"=w507:errorcluster, "Data Output Array"=w506:dbl[][])  [unwired: 3 in]
                  "Latchup Output Data" <- w506
                  n130 = call "DataFileNode_Entry_V2.vi"("error in (no error)"=w507, "Data Output Array"=w506, "Byte Stream File in"=w505) -> ("error out"=w504:errorcluster, "Byte Stream File out"=w500:refnum<file>)  [unwired: 7 in]
                  n131 = call "SupplementalDataFileNode_Entry_V2.vi"("error in (no error)"=w504, "actual count"=w501, "Byte Stream File in"=w502) -> ("error out"=w503:errorcluster, "Byte Stream File out"=w499:refnum<file>)  [unwired: 7 in]
                }
              }
              frame Enabled {
                # "Ignore this enable structure"
                n132 = disable-structure shown="Enabled" {
                  disable-tunnel: w520 -> [w528 w542 w553]
                  disable-tunnel: w519 -> [w527 w541 w554]
                  disable-tunnel: w518 -> [w526 w550 w556]
                  disable-tunnel: [w525 w542 w551] -> w517
                  disable-tunnel: [w524 w541 w552] -> w516
                  disable-tunnel: [w523 w540 w557] -> w515
                  disable-tunnel: w514 -> [w522 w547 w555]
                  frame Disabled {
                    # "DON'T Focus on this enable structure"
                    n133 = Unbundle(w522) -> (w521)
                    n134 = for {
                      tunnel: w521 -> [w536]
                      tunnel: w528 -> [w538] mode=indexing
                      tunnel: w527 -> [w537] mode=indexing
                      tunnel: [w534] -> w525 mode=indexing
                      tunnel: [w533] -> w524 mode=indexing
                      shift-right: [w532] -> w523
                      shift-left: w526 -> [w535]
                      n135 = Array Size(array=w536) -> (size(s)=w531:i32)
                      n136 = call "DataFileNode_Entry_V2.vi"("error in (no error)"=w535, "Data Output Array"=w536, "Byte Stream File in"=w538) -> ("error out"=w539:errorcluster, "Byte Stream File out"=w534:refnum<file>)  [unwired: 7 in]
                      n137 = Index Array(array=w531, index=1) -> (element=w529)
                      n138 = call "SupplementalDataFileNode_Entry_V2.vi"("error in (no error)"=w539, "actual count"=w529, "Byte Stream File in"=w537) -> ("error out"=w532:errorcluster, "Byte Stream File out"=w533:refnum<file>)  [unwired: 7 in]
                    }
                  }
                  frame Disabled {
                    # "initially thought it would be i^2, but it is i^3"
                    # "structure where all channels are in a 3 dimensional array and one file"
                    n139 = Index Array(array=w542, index=0) -> (element=w543:refnum<file>)
                    n140 = Index Array(array=w541, index=0) -> (element=w544:refnum<file>)
                    n141 = call "DataFileNode_Entry_V3.vi"("error in (no error)"=w550, "remaining elements"=w547, "Byte Stream File in"=w543) -> ("error out"=w549:errorcluster)  [unwired: 7 in, 1 out]
                    n142 = Array Size(array=w547) -> (size(s)=w548:i32)
                    n143 = call "SupplementalDataFileNode_Entry_V3.vi"("error in (no error)"=w549, "actual count"=w548, "Byte Stream File in"=w544) -> ("error out"=w540:errorcluster)  [unwired: 7 in, 1 out]
                  }
                  frame Enabled {
                    # "structure where each channel has its own data and supplemental file. Intent for faster data reading speeds in post processing. Probably not since would be i^3, but if we used multiple cores, maybe it would be advantageous"
                    n144 = for {
                      shift-right: [w559] -> w557
                      shift-left: w556 -> [w560]
                      tunnel: w555 -> [w570]
                      tunnel: w554 -> [w567] mode=indexing
                      tunnel: w553 -> [w566] mode=indexing
                      tunnel: [w565] -> w552 mode=indexing
                      tunnel: [w558] -> w551 mode=indexing
                      i -> [w564]
                      n145 = for {
                        tunnel: w570 -> [w579] mode=indexing
                        tunnel: w564 -> [w576]
                        tunnel: [w572] -> w563 mode=concatenating
                        tunnel: [w575] -> w569
                        tunnel: w567 -> [w573]
                        tunnel: w566 -> [w574]
                        tunnel: [w574] -> w561
                        tunnel: [w573] -> w565
                        tunnel: [w571] -> w568 mode=concatenating
                        n146 = Unbundle(w579) -> ("Array of fetched data"=w578:dbl[][][], "Channel Names Array"=w577:string[])  [unwired: 4 out]
                        n147 = Index Array(array=w577, index=w576) -> (element=w575:string)
                        n148 = Index Array(array=w578, index (dim 0)=w576) -> (element=w572:dbl[][])  [unwired: 2 in]
                        n149 = Array Size(array=w572) -> (size(s)=w571:i32[])
                      }
                      n150 = Bundle("Array of fetched data"=w563, w569, w568) -> (w562:T1)  [unwired: 1 in]
                      "data going into the binary file" <- w562
                      n151 = call "DataFileNode_Entry_V4.vi"("error in (no error)"=w560, "Queued Elements"=w562, "Byte Stream File in"=w561) -> ("error out"=w559:errorcluster, "Byte Stream File out"=w558:refnum<file>)  [unwired: 7 in]
                    }
                  }
                }
              }
            }
          }
        }
        n152 = local read "Exiting"() -> (w421:bool)
        n153 = Equal To 0?(x=w412) -> (x = 0?=w420:bool)
        n154 = And(x=w420, y=w421) -> (x .and. y?=w419:bool)
      }
      n155 = disable-structure shown="Enabled" {
        disable-tunnel: _ -> [w407 _]
        disable-tunnel: w390 -> [w406 w408]
        disable-tunnel: [w405 w408] -> w389
        disable-tunnel: w388 -> [w404 _]
        frame Disabled {
          n156 = Index Array(array=w404, index (row)=0 ("index")) -> (element=w402:refnum<file>[])  [unwired: 1 in]
          n157 = call "DataFileNode_Entry_V5.vi"("error in (no error)"=w406, "Data to be inputter"=w407, "Byte Stream File in"=w402) -> ("error out"=w405:errorcluster)  [unwired: 7 in, 1 out]
        }
        frame Enabled {
          (unwired) T1 {"Array of fetched data"=[], "", []} ("cluster")
        }
      }
      "DCPowerInformationClusterArray_Input 2" <- w392
    }
    frame Disabled {
    }
  }
  n158 = for {
    tunnel: w49 -> [w584] mode=indexing
    tunnel: w48 -> [w582] mode=indexing
    shift-right: [w580] -> w46
    shift-left: w47 -> [w583]
    n159 = Close File(refnum=w584, error in=w583) -> (error out=w581:errorcluster)  [unwired: 1 out]
    n160 = Close File(refnum=w582, error in=w581) -> (error out=w580:errorcluster)  [unwired: 1 out]
  }
  n161 = Merge Errors(w51, w46) -> (w25:errorcluster)
  n162 = disable-structure shown="Disabled" {
    frame Disabled {
      n163 = To Double Precision Float() -> (double precision float=w589:dbl)  [unwired: 1 in]
      n164 = To Double Precision Float() -> (double precision float=w590:dbl)  [unwired: 1 in]
      n165 = Subtract(x=w589, y=w590) -> (x-y=w588:dbl)
      n166 = Greater?(x=w588, y=10.0) -> (0:w587:bool)
      n167 = case shown="False" w587 {
        tunnel: [w591 w597] -> w586
        tunnel: [w592 w594] -> _
        tunnel: _ -> [w592 _]
        tunnel: [w591 w593] -> _
        frame False {
        }
        frame True {
          n168 = Get Date/Time In Seconds() -> (seconds since 1Jan1904=w594:timestamp)
          n169 = property on="Voltage 2" class="WFChart (strict)" props=["History Data", "XScale", "ScaleFit", "XScale", "Minimum", "XScale", "Maximum"](error in=w597, "History Data"=waveform(dbl)[][] []) -> (error out=w595:errorcluster)  [unwired: 4 in, 1 out]
          n170 = property on="Current 2" class="WFChart (strict)" props=["History Data", "XScale", "ScaleFit", "XScale", "Minimum", "XScale", "Maximum"](error in=w595) -> (error out=w593:errorcluster)  [unwired: 5 in, 1 out]
        }
      }
    }
    frame Enabled {
    }
  }
  n171 = Unbundle(w21) -> ("created path array"=w5:path[])  [unwired: 2 out]
  n172 = case shown="True" w10 {
    selector: w10 -> [w601 w633]
    tunnel: w25 -> [w600 w644]
    tunnel: [w600 w627] -> w24
    tunnel: [w606 w643] -> w20
    tunnel: w19 -> [w606 w642]
    tunnel: [w605 w641] -> w18
    tunnel: w17 -> [w605 w640]
    tunnel: [w604 w639] -> w16
    tunnel: w15 -> [w604 w638]
    tunnel: [w603 w637] -> w14
    tunnel: w13 -> [w603 w636]
    tunnel: [w602 w635] -> w12
    tunnel: w11 -> [w602 w634]
    tunnel: [w601 w633] -> w9
    tunnel: [string[][][] [] w632] -> w8
    tunnel: [string[][] [] ("DCPowerInfoArray") w622] -> w7
    tunnel: w5 -> [_ w625]
    frame False {
    }
    frame True {
      n173 = for {
        shift-right: [w646] -> w628
        shift-left: w644 -> [w658]
        tunnel: w634 -> [w649] mode=indexing
        shift-right: [w657] -> w643
        shift-left: w642 -> [w657]
        shift-right: [w656] -> w641
        shift-left: w640 -> [w656]
        shift-right: [w655] -> w639
        shift-left: w638 -> [w655]
        shift-right: [w654] -> w637
        shift-left: w636 -> [w654]
        shift-right: [w653] -> w635
        shift-left: w634 -> [w653]
        tunnel: [w645] -> w632 mode=indexing
        shift-right: [w651] -> w622
        shift-left: string[][] [] ("DCPowerInfoArray") -> [w652]
        # "This puts all the instruments together in one output"
        n174 = Unbundle(w649) -> ("instrument handle out"=w660:refnum<k15>, w659:string)  [unwired: 5 out]
        n175 = call <instrlib>:"niDCPower Abort With Channels.vi"("error in (no error)"=w658, "channel name"=w659, "instrument handle"=w660) -> ("error out"=w647:errorcluster)  [unwired: 7 in, 1 out]
        n176 = call "DCPower_ParameterCreation.vi"("error in"=w647, "Precision"="8", "DCPowerInformationByInstrument"=w649) -> ("error out"=w646:errorcluster, "DCPowerInfoArray"=w645:string[][])
        n177 = Insert Into Array(array=w652, index (col)=0 ("disabled index (col)"), new element=w645) -> (w651:string[][])  [unwired: 1 in]
      }
      n178 = Concatenate Strings("Channel Name " ("string")) -> (w617:string)
      n179 = Concatenate Strings("Voltage (V) " ("string")) -> (w619:string)
      n180 = Concatenate Strings("Measure Record delta Time (s) " ("string")) -> (w621:string)
      n181 = Concatenate Strings("Instrument Name " ("string")) -> (w616:string)
      n182 = Concatenate Strings("Instrument Channel Number " ("string")) -> (w618:string)
      n183 = Concatenate Strings("Current Limit (A) " ("string")) -> (w620:string)
      n184 = Build Array(w616, w617, w618, w619, w620, w621) -> (w609:string[])
      n185 = Insert Into Array(array=w622, index (col)=0 ("disabled index (col)"), new element=w609) -> (w608:string[][])  [unwired: 1 in]
      n186 = Build Path(base path=w625, name or relative path="DCPOW_Params.csv") -> (appended path=w626:path)
      n187 = call-poly <vilib>:"Write Delimited Spreadsheet.vi"("file path (dialog if empty)"=w626, "format (%s)"="%s" ("format (%.3f)"), "2D data"=w608, "error in (no error)"=w628, "transpose? (no:F)"=TRUE, "delimiter (\\t)"="," ("delimiter (\\t)")) -> ("error out"=w627:errorcluster)  [unwired: 8 in, 1 out]
    }
  }
  "DCPowerInformationClusterArray_Output" <- w12
  "VISAPowerInfoInputOutput" <- w14
  "Run Data SubPanel Output" <- w16
  "RF Block Parameters Output" <- w18
  "Oscilloscope Info Array Output" <- w20
  "Data Was Collected?" <- w9
  "Array" <- w8
  "DCPowerInfoArray" <- w7
  n188 = List Folder(path=w5, pattern="*.txt", error in=w24) -> (path out=w30:path, filenames=w29:string[], error out=w28:errorcluster)  [unwired: 1 in, 1 out]
  n189 = for {
    tunnel: [w661] -> w31
    tunnel: w30 -> [w661]
    tunnel: w29 -> [w663] mode=indexing
    shift-right: [w664] -> w27
    shift-left: w28 -> [w665]
    n190 = Build Path(base path=w661, name or relative path=w663) -> (appended path=w662:path)
    n191 = Delete(path (use dialog)=w662, error in=w665) -> (error out=w664:errorcluster)  [unwired: 3 in, 2 out]
  }
  n192 = Strip Path(path=w31) -> (name=w35:string)  [unwired: 1 out]
  n193 = Concatenate Strings(w35, "_DCPOWER_COPYFOLDER" ("name or relative path")) -> (w33:string)
  n194 = Build Path(base path=w31, name or relative path=w33) -> (appended path=w42:path)
  n195 = Create Folder(path (use dialog)=w42, error in=w27) -> (created path=w37:path, error out=w40:errorcluster)  [unwired: 1 in, 1 out]
  n196 = List Folder(path=w31, error in=w40) -> (path out=w39:path, filenames=w38:string[], error out=w36:errorcluster)  [unwired: 2 in, 1 out]
  n197 = for {
    tunnel: w39 -> [w671]
    tunnel: w38 -> [w670] mode=indexing
    tunnel: w37 -> [w666]
    shift-right: [w673] -> w41
    shift-left: w36 -> [w667]
    tunnel: [w666] -> _
    n198 = Build Path(base path=w671, name or relative path=w670) -> (appended path=w668:path)
    n199 = Build Path(base path=w666, name or relative path=w670) -> (appended path=w669:path)
    n200 = Copy(8:w667, 9:TRUE ("overwrite (F)"), 10:w669, 11:w668) -> (0:w673:errorcluster)  [unwired: 1 in, 2 out]
  }
  "error out" <- w41
